vi "Cleanup.vi"(8 "error in (no error)":errorcluster, 11 "Controller in":refnum<class "Controller.lvclass">) -> (0 "error out":errorcluster)   [LabVIEW 2020, in "Controller.lvclass"]
uses:
  Controller.lvclass
  Controller.lvclass/Controller.ctl
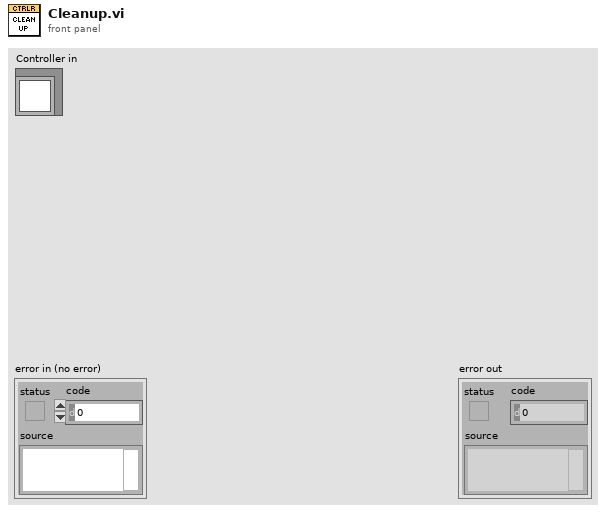
[diagram p1: front panel]
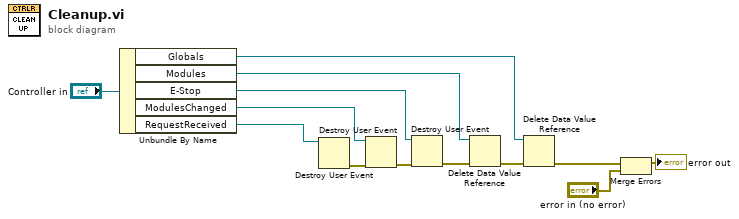
[diagram p0: block diagram]
diagram:
  n1 = Unbundle By Name("Controller in") -> ("Globals"=w12:refnum<data-value>, "Modules"=w10:refnum<data-value>, "E-Stop"=w4:refnum<user-event>, "ModulesChanged"=w5:refnum<user-event>, "RequestReceived"=w6:refnum<user-event>)
  n2 = Destroy User Event(user event=w6) -> (error out=w7:errorcluster)  [unwired: 1 in]
  n3 = Destroy User Event(user event=w5, error in=w7) -> (error out=w8:errorcluster)
  n4 = Destroy User Event(user event=w4, error in=w8) -> (error out=w3:errorcluster)
  n5 = Delete Data Value Reference(data value reference=w10, error in=w3) -> (error out=w11:errorcluster)  [unwired: 1 out]
  n6 = Delete Data Value Reference(data value reference=w12, error in=w11) -> (error out=w1:errorcluster)  [unwired: 1 out]
  n7 = Merge Errors(w1, "error in (no error)") -> (→"error out":errorcluster)
